vi "VariableGlobal.vi"() -> ()   [LabVIEW 2020]
panel:
  out "initialized array":dbl[](array[numeric])
  in  "Thermometer":dbl(slide) scale=0.0..100.0
  out "String":string
  in  "Boolean 3":bool
  out "Boolean 2":bool
  in  "Boolean":bool
  in  "stop":bool
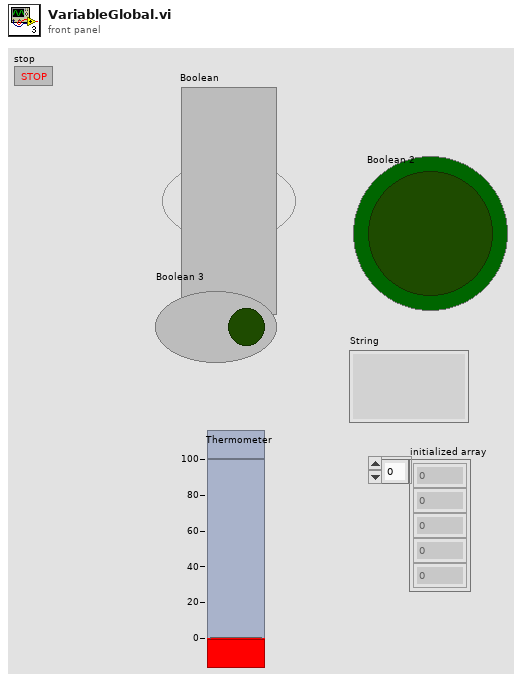
[diagram p1: front panel]
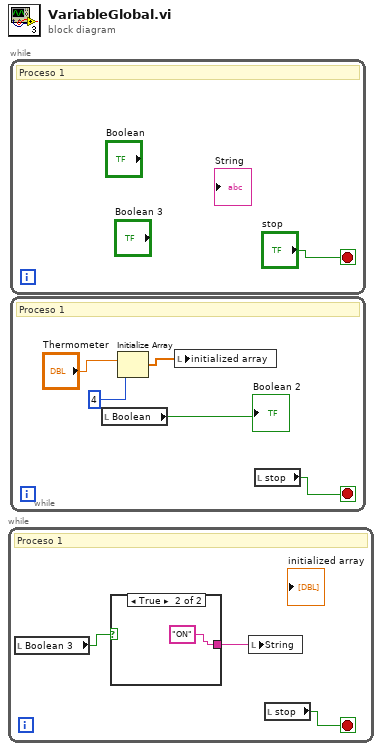
[diagram p0: block diagram]
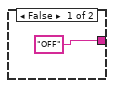
[diagram p2: hidden frame]
diagram:
  n1 = while {
    stop <- w3 stop-if-true
    # "Proceso 1"
    n2 = local read "Boolean 3"() -> (w2:bool)
    n3 = case shown="True" w2 {
      tunnel: ["OFF" "ON"] -> w1
      frame False {
      }
      frame True {
      }
    }
    n4 = local write "String"(w1) -> ()
    n5 = local read "stop"() -> (w3:bool)
  }
  n6 = while {
    stop <- "stop" stop-if-true
    # "Proceso 1"
  }
  n7 = while {
    stop <- w11 stop-if-true
    # "Proceso 1"
    n8 = local read "Boolean"() -> (→"Boolean 2":bool)
    n9 = Initialize Array("Thermometer", 4 ("dimension size")) -> (w7:dbl[])
    n10 = local write "initialized array"(w7) -> ()
    n11 = local read "stop"() -> (w11:bool)
  }
